vi "autoqueue_dual.vi"(0 "cluster":T3, 1 "output cluster":T2, 3 "Cluster":cluster{"1":bool, "2":bool}, 5 "1to4":T1, 7 "path":bool, 9 "Str Refnum":refnum<vi>, 11 "error out":errorcluster, 12 "Slide Refnum":refnum<vi>, 13 "Report Data.Degree":dbl[][](array[numeric]), 14 "Slide Refnum 2":refnum<vi>) -> (15 "error out 2":errorcluster)   [LabVIEW 2015]
uses:
  Typedef/Inst. Queue.ctl
  Typedef/State.ctl
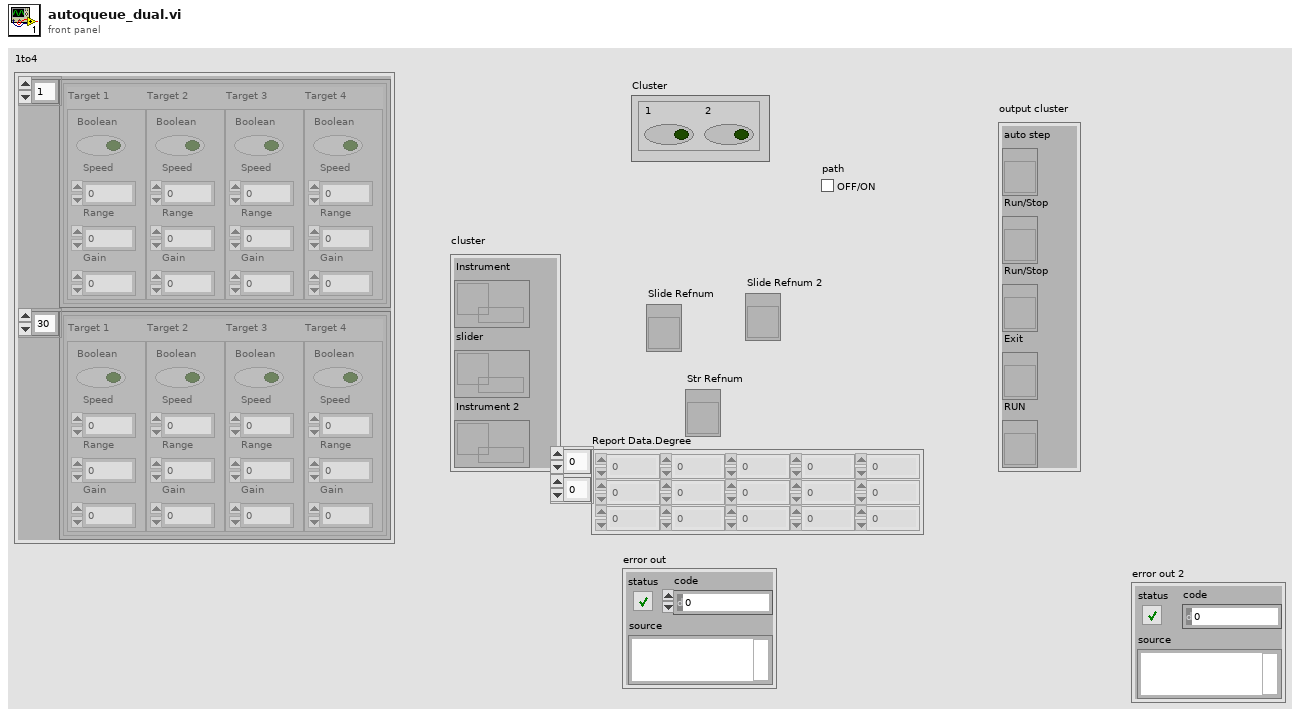
[diagram p1: front panel]
types:
  T1 = cluster{cluster{"Target 1":cluster{"Boolean":bool, "Speed":dbl, "Range":dbl, "Gain":dbl}, "Target 2":cluster{"Boolean":bool, "Speed":dbl, "Range":dbl, "Gain":dbl}, "Target 3":cluster{"Boolean":bool, "Speed":dbl, "Range":dbl, "Gain":dbl}, "Target 4":cluster{"Boolean":bool, "Speed":dbl, "Range":dbl, "Gain":dbl}}[], cluster{"Target 1":cluster{"Boolean":bool, "Speed":dbl, "Range":dbl, "Gain":dbl}, "Target 2":cluster{"Boolean":bool, "Speed":dbl, "Range":dbl, "Gain":dbl}, "Target 3":cluster{"Boolean":bool, "Speed":dbl, "Range":dbl, "Gain":dbl}, "Target 4":cluster{"Boolean":bool, "Speed":dbl, "Range":dbl, "Gain":dbl}}[]}
  T2 = cluster{"auto step":refnum<vi>, "Run/Stop":refnum<vi>, "Run/Stop":refnum<vi>, "Exit":refnum<vi>, "RUN":refnum<vi>}
  T3 = cluster{"Instrument":refnum<queue>, "slider":refnum<queue>, "Instrument 2":refnum<queue>}
  T4 = cluster{"Target 1":cluster{"Boolean":bool, "Speed":dbl, "Range":dbl, "Gain":dbl}, "Target 2":cluster{"Boolean":bool, "Speed":dbl, "Range":dbl, "Gain":dbl}, "Target 3":cluster{"Boolean":bool, "Speed":dbl, "Range":dbl, "Gain":dbl}, "Target 4":cluster{"Boolean":bool, "Speed":dbl, "Range":dbl, "Gain":dbl}}[]
  T5 = typedef "Inst. Queue.ctl" = cluster{enum16{"auto mode", "Idle", "Inst. Connect", "£m Data", "Inst. Update", "Freq. (GHz)", "rx att", "GTX (dB)", "GRX (dB)", "Range Trim(m)", "Gain Trim (dB)", "Distance to RUT", "Mapping", "Convert", "RF ON/OFF", "Run", "Direct Program", "Stop", "Dynamic", "dyset", "Exit"}, "variant":variant}
  T6 = typedef "State.ctl" = enum16{"Idle", "Initial", "Update", "get angle", "Axis", "Connect", "Creep", "Speed", "Distance", "Move Method", "Move Mode", "Direct of Movement", "Initail Speed", "Sramp", "Normal Open", "Acceleration", "Deceleration", "Angle", "Move&Rotate", "Rotate", "Rotate_2", "Return to Origin", "Move", "Inching", "Return to Zero", "Return to Middle", "Go to Step1", "Go to Step2", "Go to Step3", "Initial to Y Step", "Select Speed", "auto mode", "Stop", "reset xy", "reset ant", "set speed", "Exit"}
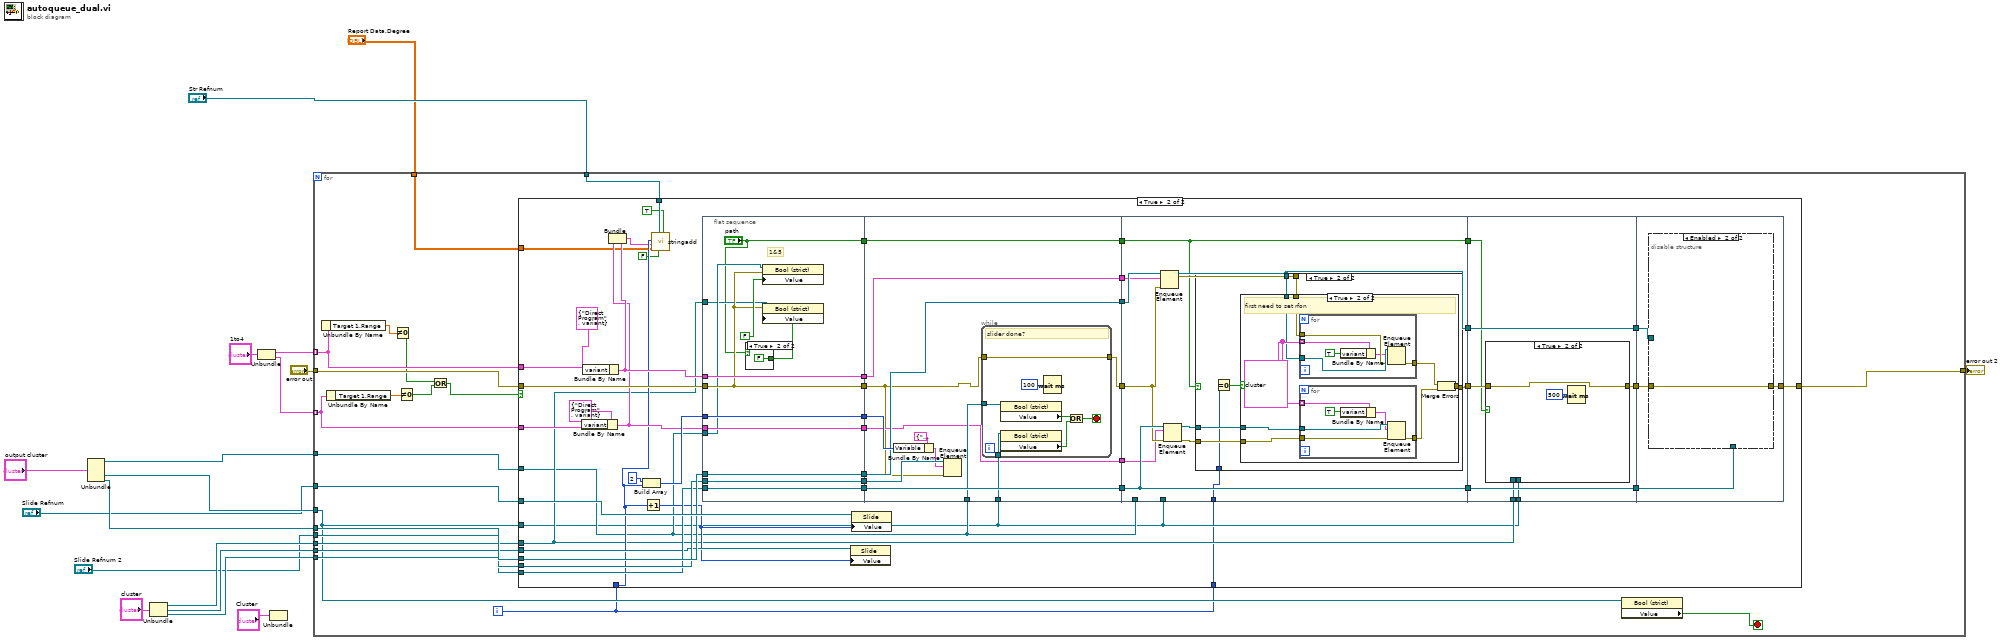
[diagram p0: block diagram]
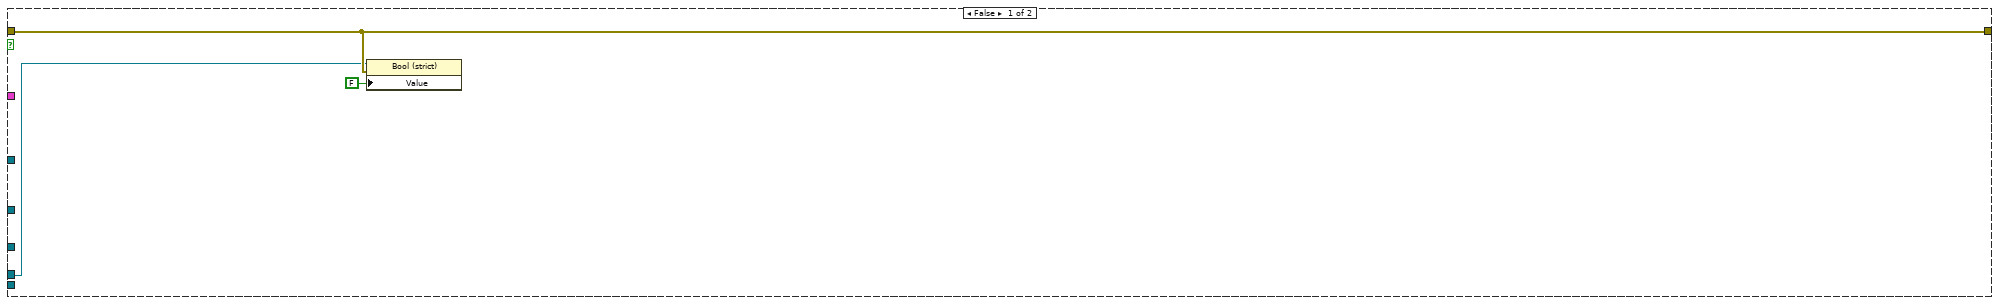
[diagram p2: hidden frame]
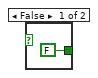
[diagram p3: hidden frame]
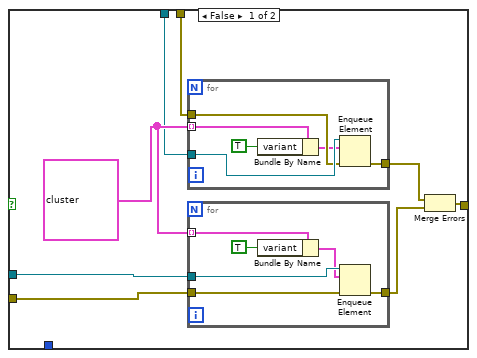
[diagram p4: hidden frame]
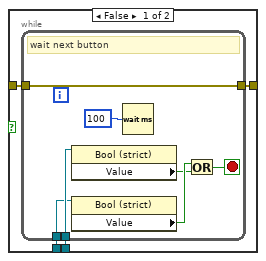
[diagram p6: hidden frame]
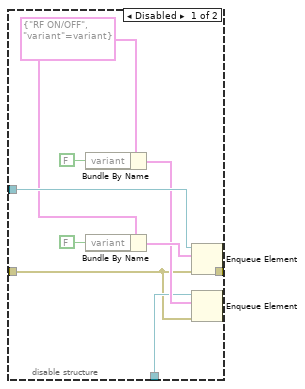
[diagram p7: hidden frame]
diagram:
  n1 = Unbundle("output cluster") -> ("auto step"=w9:refnum<vi>, "Exit"=w8:refnum<vi>, "RUN"=w10:refnum<vi>)  [unwired: 2 out]
  n2 = Unbundle("cluster") -> ("Instrument"=w16:refnum<queue>, "slider"=w15:refnum<queue>, "Instrument 2"=w7:refnum<queue>)
  n3 = Unbundle("1to4") -> (w13:T4, w2:T4)
  n4 = Unbundle("Cluster") -> ()  [unwired: 2 out]
  n5 = for {
    tunnel: w16 -> [w36]
    tunnel: w13 -> [w27] mode=indexing
    tunnel: w15 -> [w35]
    tunnel: "Slide Refnum" -> [w37]
    tunnel: w10 -> [w30]
    tunnel: w9 -> [w34]
    tunnel: w8 -> [w28]
    tunnel: w7 -> [w33]
    tunnel: "Slide Refnum 2" -> [w32]
    tunnel: "Str Refnum" -> [w31]
    tunnel: w2 -> [w26] mode=indexing
    tunnel: "error out" -> [w38]
    tunnel: [w39] -> w6
    tunnel: "Report Data.Degree" -> [w20]
    i -> [w19]
    stop <- w29 stop-if-true
    n6 = Unbundle By Name(w27) -> ("Target 1.Range"=w24:dbl)
    n7 = Unbundle By Name(w26) -> ("Target 1.Range"=w25:dbl)
    n8 = Not Equal To 0?(x=w24) -> (x != 0?=w22:bool)
    n9 = Not Equal To 0?(x=w25) -> (x != 0?=w23:bool)
    n10 = Or(x=w22, y=w23) -> (x .or. y?=w21:bool)
    n11 = case shown="True" w21 {
      tunnel: [w42 w73] -> w39
      tunnel: w38 -> [w42 w72]
      tunnel: w37 -> [_ w71]
      tunnel: w36 -> [_ w70]
      tunnel: w35 -> [_ w69]
      tunnel: w34 -> [_ w47]
      tunnel: w33 -> [_ w66]
      tunnel: w32 -> [_ w65]
      tunnel: w27 -> [_ w63]
      tunnel: w26 -> [_ w60]
      tunnel: w19 -> [_ w57]
      tunnel: w31 -> [_ w56]
      tunnel: w30 -> [w41 w54]
      tunnel: w28 -> [_ w46]
      tunnel: w20 -> [_ w48]
      tunnel: w19 -> [_ w43]
      frame False {
        n12 = property on="Property Node" class="Bool (strict)"(reference=w41, error in=w42, "Value"=FALSE) -> ()  [unwired: 2 out]
      }
      frame True {
        n13 = Bundle By Name(cluster=T5 {enum."Direct Program", "variant"=variant}, "variant"=w60) -> (w58:T5)
        n14 = Bundle By Name(cluster=T5 {enum."Direct Program", "variant"=variant}, "variant"=w63) -> (w59:T5)
        n15 = Bundle(w59, w58) -> (w55:cluster{T5, T5})  [unwired: 1 in]
        n16 = Build Array(2 ("element"), w57) -> (w67:i32[])
        n17 = Increment(x=w57) -> (x+1=w64:i32)
        n18 = call "stringadd.vi"("Report Data.Degree"=w48, "Mode"=TRUE, "s/d setting"=FALSE, "Str Refnum"=w56, "variant"=w55, "Numeric"=w57) -> ()  [unwired: 6 in]
        n19 = flat-sequence {
          tunnel: w66 -> [w97]
          tunnel: w47 -> [w93]
          tunnel: w67 -> [w98]
          tunnel: w72 -> [w95]
          tunnel: w70 -> [w99]
          tunnel: w59 -> [w100]
          tunnel: w69 -> [w101]
          tunnel: [w101] -> w89
          tunnel: [w100] -> w88
          tunnel: [w99] -> w87
          tunnel: [w95] -> w86
          tunnel: [w98] -> w85
          tunnel: [w97] -> w84
          tunnel: w58 -> [w94]
          tunnel: [w94] -> w83
          tunnel: w54 -> [w92]
          tunnel: ["path"] -> w50
          tunnel: [w110] -> w82
          tunnel: [w107] -> w81
          tunnel: [w112] -> w80
          tunnel: w89 -> [w116]
          tunnel: w88 -> [w106]
          tunnel: w87 -> [w107]
          tunnel: w86 -> [w104]
          tunnel: w85 -> [w114]
          tunnel: w84 -> [w112]
          tunnel: w83 -> [w105]
          tunnel: [w111] -> w51
          tunnel: w50 -> [w111]
          tunnel: w47 -> [w109]
          tunnel: w46 -> [w108]
          tunnel: [w106] -> w45
          tunnel: [w105] -> w44
          tunnel: w82 -> [w129]
          tunnel: [w135] -> w79
          tunnel: [w133] -> w78
          tunnel: w81 -> [w134]
          tunnel: w47 -> [_]
          tunnel: [w131] -> w77
          tunnel: w80 -> [w131]
          tunnel: w46 -> [_]
          tunnel: [w125] -> w52
          tunnel: w51 -> [w125]
          tunnel: w45 -> [w127]
          tunnel: w44 -> [w126]
          tunnel: w43 -> [w124]
          tunnel: w79 -> [w190]
          tunnel: [w189] -> w76
          tunnel: [w188] -> w75
          tunnel: w78 -> [w188]
          tunnel: [w187] -> w74
          tunnel: w77 -> [w187]
          tunnel: w46 -> [w186]
          tunnel: w54 -> [w185]
          tunnel: w52 -> [w184]
          tunnel: [w207] -> w73
          tunnel: w76 -> [w204]
          tunnel: w75 -> [w206]
          tunnel: w74 -> [w205]
          frame #0 {
            # "1&5"
            n20 = case shown="True" "path" {
              tunnel: [FALSE FALSE] -> w91
              frame False {
              }
              frame True {
              }
            }
            n21 = property on="Property Node" class="Bool (strict)"(reference=w93, error in=w95, "Value"=FALSE) -> ()  [unwired: 2 out]
            n22 = property on="Property Node" class="Bool (strict)"(reference=w92, error in=w95, "Value"=w91) -> ()  [unwired: 2 out]
          }
          frame #1 {
            n23 = Bundle By Name(cluster=cluster{"State":T6, "Variable":variant} {"State"=enum."auto mode", "Variable"=variant}, "Variable"=w114) -> (w113:cluster{"State":T6, "Variable":variant})
            n24 = Enqueue Element(queue=w116, element=w113, error in (no error)=w104) -> ()  [unwired: 1 in, 3 out]
            n25 = while {
              tunnel: w104 -> [w123]
              tunnel: [w123] -> w110
              tunnel: w109 -> [w118]
              tunnel: w108 -> [w117]
              stop <- w119 stop-if-true
              # "slider done?"
              n26 = property on="Property Node" class="Bool (strict)"(reference=w118) -> ("Value"=w121:bool)  [unwired: 1 in, 2 out]
              n27 = property on="Property Node" class="Bool (strict)"(reference=w117) -> ("Value"=w120:bool)  [unwired: 1 in, 2 out]
              n28 = Wait (ms)(milliseconds to wait=u32 100) -> ()  [unwired: 1 out]
              n29 = Or(x=w121, y=w120) -> (x .or. y?=w119:bool)
            }
          }
          frame #2 {
            n30 = Enqueue Element(queue=w134, element=w127, error in (no error)=w129) -> (queue out=w133:refnum<queue>, error out=w132:errorcluster)  [unwired: 1 in, 1 out]
            n31 = Enqueue Element(queue=w131, element=w126, error in (no error)=w129) -> (queue out=w130:refnum<queue>, error out=w128:errorcluster)  [unwired: 1 in, 1 out]
            n32 = case shown="True" w125 {
              tunnel: [w140 w162] -> w135
              tunnel: w133 -> [w139 w161]
              tunnel: w132 -> [w138 w160]
              tunnel: w130 -> [w137 w159]
              tunnel: w128 -> [w136 w158]
              tunnel: w124 -> [_ w157]
              frame False {
                w143 = T5[] [{enum."Convert", "variant"=variant}, {enum."RF ON/OFF", "variant"=variant}]
                n33 = for {
                  tunnel: w143 -> [w146] mode=indexing
                  tunnel: w139 -> [w149]
                  tunnel: w138 -> [w148]
                  tunnel: [w147] -> w142
                  n34 = Bundle By Name(cluster=w146, "variant"=TRUE) -> (w145:T5)
                  n35 = Enqueue Element(queue=w149, element=w145, error in (no error)=w148) -> (error out=w147:errorcluster)  [unwired: 1 in, 2 out]
                }
                n36 = for {
                  tunnel: w143 -> [w152] mode=indexing
                  tunnel: w137 -> [w155]
                  tunnel: w136 -> [w154]
                  tunnel: [w153] -> w141
                  n37 = Bundle By Name(cluster=w152, "variant"=TRUE) -> (w151:T5)
                  n38 = Enqueue Element(queue=w155, element=w151, error in (no error)=w154) -> (error out=w153:errorcluster)  [unwired: 1 in, 2 out]
                }
                n39 = Merge Errors(w142, w141) -> (w140:errorcluster)
              }
              frame True {
                n40 = Equal To 0?(x=w157) -> (x = 0?=w156:bool)
                n41 = case shown="True" w156 {
                  tunnel: [w163 w168] -> w162
                  tunnel: w161 -> [_ w167]
                  tunnel: w160 -> [_ w166]
                  tunnel: w159 -> [_ w165]
                  tunnel: w158 -> [w163 w164]
                  frame False {
                    # "others don't need set rfon"
                  }
                  frame True {
                    w171 = T5[] [{enum."Convert", "variant"=variant}, {enum."RF ON/OFF", "variant"=variant}]
                    # "first need to set rfon"
                    n42 = for {
                      tunnel: w171 -> [w180] mode=indexing
                      tunnel: w167 -> [w183]
                      tunnel: w166 -> [w182]
                      tunnel: [w181] -> w170
                      n43 = Bundle By Name(cluster=w180, "variant"=TRUE) -> (w179:T5)
                      n44 = Enqueue Element(queue=w183, element=w179, error in (no error)=w182) -> (error out=w181:errorcluster)  [unwired: 1 in, 2 out]
                    }
                    n45 = for {
                      tunnel: w171 -> [w174] mode=indexing
                      tunnel: w165 -> [w177]
                      tunnel: w164 -> [w176]
                      tunnel: [w175] -> w169
                      n46 = Bundle By Name(cluster=w174, "variant"=TRUE) -> (w173:T5)
                      n47 = Enqueue Element(queue=w177, element=w173, error in (no error)=w176) -> (error out=w175:errorcluster)  [unwired: 1 in, 2 out]
                    }
                    n48 = Merge Errors(w170, w169) -> (w168:errorcluster)
                  }
                }
              }
            }
          }
          frame #3 {
            n49 = case shown="True" w184 {
              tunnel: w190 -> [w194 w202]
              tunnel: [w193 w202] -> w189
              tunnel: w186 -> [w192 _]
              tunnel: w185 -> [w191 _]
              frame False {
                n50 = while {
                  tunnel: w194 -> [w200]
                  tunnel: [w200] -> w193
                  tunnel: w192 -> [w196]
                  tunnel: w191 -> [w195]
                  stop <- w197 stop-if-true
                  # "wait next button"
                  n51 = property on="Property Node" class="Bool (strict)"(reference=w196) -> ("Value"=w198:bool)  [unwired: 1 in, 2 out]
                  n52 = property on="Property Node" class="Bool (strict)"(reference=w195) -> ("Value"=w199:bool)  [unwired: 1 in, 2 out]
                  n53 = Wait (ms)(milliseconds to wait=u32 100) -> ()  [unwired: 1 out]
                  n54 = Or(x=w199, y=w198) -> (x .or. y?=w197:bool)
                }
              }
              frame True {
                n55 = Wait (ms)(milliseconds to wait=u32 500) -> ()  [unwired: 1 out]
              }
            }
          }
          frame #4 {
            n56 = disable-structure shown="Enabled" {
              disable-tunnel: [w216 w217] -> w207
              disable-tunnel: w206 -> [w215 _]
              disable-tunnel: w205 -> [w211 _]
              disable-tunnel: w204 -> [w210 w217]
              frame Disabled {
                w208 = T5 {enum."RF ON/OFF", "variant"=variant}
                n57 = Bundle By Name(cluster=w208, "variant"=FALSE) -> (w212:T5)
                n58 = Bundle By Name(cluster=w208, "variant"=FALSE) -> (w214:T5)
                n59 = Enqueue Element(queue=w215, element=w214, error in (no error)=w210) -> (error out=w216:errorcluster)  [unwired: 1 in, 2 out]
                n60 = Enqueue Element(queue=w211, element=w212, error in (no error)=w210) -> ()  [unwired: 1 in, 3 out]
              }
              frame Enabled {
              }
            }
          }
        }
        n61 = property class="Slide"(reference=w65, "Value"=w64) -> ()  [unwired: 1 in, 2 out]
        n62 = property class="Slide"(reference=w71, "Value"=w64) -> ()  [unwired: 1 in, 2 out]
      }
    }
    n63 = property on="Property Node" class="Bool (strict)"(reference=w28) -> ("Value"=w29:bool)  [unwired: 1 in, 2 out]
  }
  "error out 2" <- w6
